vi "rsa_decryptor.vi"(1 "Encrypted text":string="HALLO", 2 "Own module":string="HALLO", 3 "Own private key":string="HALLO") -> (0 "Decrypted text":string="HALLO")   [LabVIEW 2017]
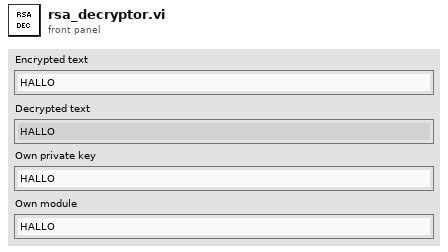
[diagram p1: front panel]
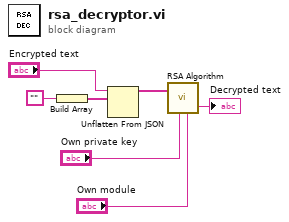
[diagram p0: block diagram]
diagram:
  n1 = Build Array("") -> (w3:string[])
  n2 = Unflatten From JSON(JSON string="Encrypted text", type and defaults=w3) -> (value=w1:string[])  [unwired: 5 in, 1 out]
  n3 = call "RSA Algorithm.vi"("Exponent"="Own private key", "Modulo"="Own module", "Ciphertext"=w1) -> ("Output"=→"Decrypted text":string)  [unwired: 3 in, 1 out]
